vi "Initialize.vi"(8 "error in (no error)":errorcluster, 9 "settings":T1[](array[typedef]), 10 "Group Configurations":refnum<class "Group Configuration.lvclass">[](array[class]), 11 "Type Converter in":refnum<class "Default Buffer Converter.lvclass">) -> (0 "error out":errorcluster, 3 "Type Converter out":refnum<class "Default Buffer Converter.lvclass">)   [LabVIEW 2017, in "DSF Core.lvlib" / "Default Buffer Converter.lvclass"]
uses:
  Default Buffer Converter.lvclass
  Classes/Configuration/Core/Group/Group Configuration.lvclass
  Typedefs/DSF Settings Info.ctl
  Conversion.ctl
  Conversion Block.ctl
  Typedefs/DSF Data Type.ctl
  Default Buffer Converter.lvclass/Default Buffer Converter.ctl
  Classes/Configuration/Core/Transfer/Transfer Configuration.lvclass
  DSF Core.lvlib
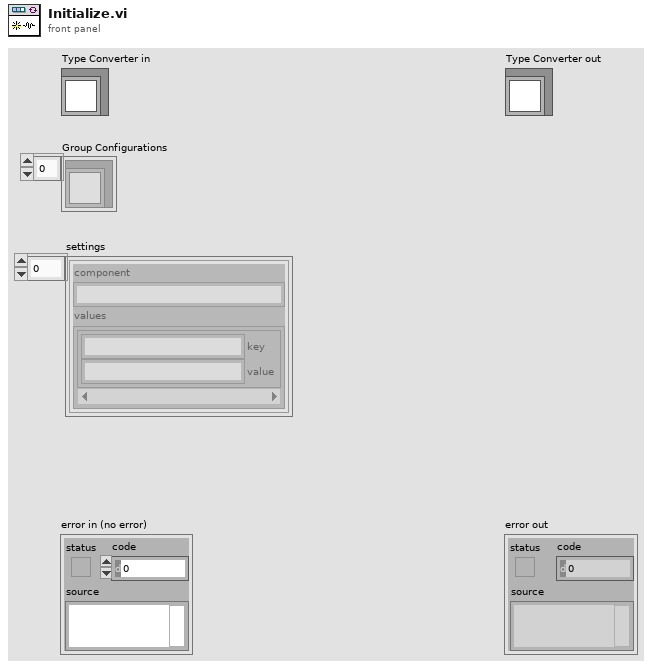
[diagram p1: front panel]
types:
  T1 = typedef "DSF Core.lvlib/DSF Settings Info.ctl" = cluster{"component":string, "values":cluster{"key":string, "value":string}[]}
  T2 = typedef "DSF Core.lvlib/Default Buffer Converter.lvclass/Conversion.ctl" = cluster{"conversion blocks":T3[]}
  T3 = typedef "DSF Core.lvlib/Default Buffer Converter.lvclass/Conversion Block.ctl" = cluster{"engine offset":u64, "engine data type":T4, "string offset":u64, "string data type":T4, "engine byte order":enum16{"big-endian, network order", "native, host order", "little-endian"}, "string byte order":enum16{"big-endian, network order", "native, host order", "little-endian"}, "count":u64}
  T4 = typedef "DSF Core.lvlib/DSF Data Type.ctl" = enum8{"Bool", "SGL", "DBL", "I8", "I16", "I32", "I64", "U8", "U16", "U32", "U64"}
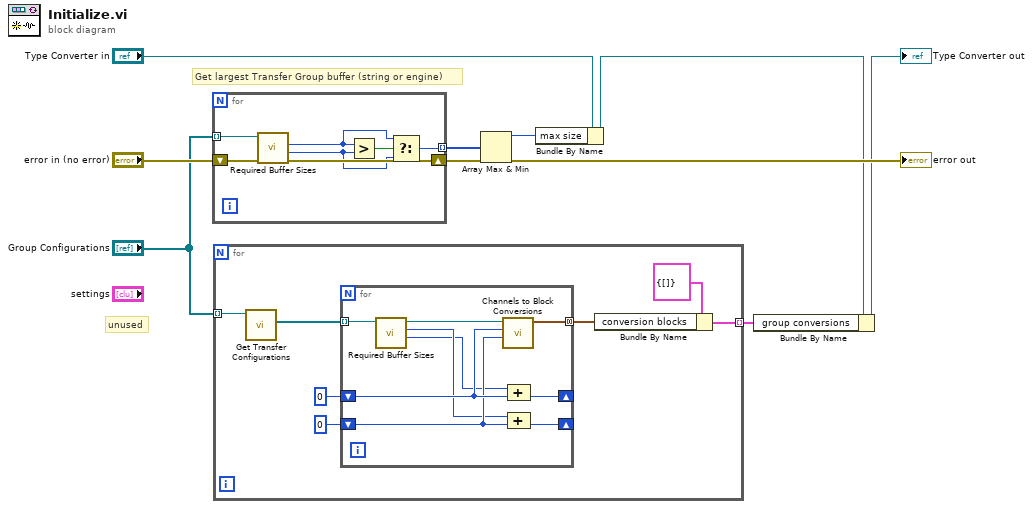
[diagram p0: block diagram]
diagram:
  # "Get largest Transfer Group buffer (string or engine)"
  # "unused"
  n1 = for {
    tunnel: "Group Configurations" -> [w14] mode=indexing
    tunnel: [w15] -> w8 mode=indexing
    shift-right: [w12] -> w9
    shift-left: "error in (no error)" -> [w13]
    n2 = call-dynamic "Required Buffer Sizes.vi"("error in (no error)"=w13, "Group Configuration in"=w14) -> ("error out"=w12:errorcluster, "string size"=w11:u64, "engine size"=w10:u64)  [unwired: 6 in, 1 out]
    n3 = Greater?(x=w10, y=w11) -> (0:w16:bool)
    n4 = Select(t=w10, s=w16, f=w11) -> (s? t:f=w15:u64)
  }
  "error out" <- w9
  n5 = for {
    tunnel: "Group Configurations" -> [w18] mode=indexing
    tunnel: [w21] -> w6 mode=indexing
    n6 = call "Get Transfer Configurations.vi"("Group Configuration in"=w18) -> ("Transfer Configurations"=w17:refnum<class "Transfer Configuration.lvclass">[])  [unwired: 8 in, 2 out]
    n7 = for {
      tunnel: w17 -> [w27] mode=indexing
      tunnel: [w32] -> w22 mode=concatenating
      shift-right: [w31] -> _
      shift-left: u64 0 ("engine buffer size") -> [w29]
      shift-right: [w30] -> _
      shift-left: u64 0 ("engine buffer size") -> [w28]
      n8 = call-dynamic "Required Buffer Sizes.vi"("Transfer Configuration in"=w27) -> ("string size"=w24:u64, "engine size"=w25:u64, "Transfer Configuration out"=w26:refnum<class "Transfer Configuration.lvclass">)  [unwired: 7 in, 1 out]
      n9 = call "Channels to Block Conversions.vi"("initial engine buffer offset"=w28, "initial string buffer offset"=w29, "Transfer Configuration"=w26) -> ("Transfer conversion descriptors"=w32:T3[])  [unwired: 8 in]
      n10 = Compound Arithmetic op=ADD(w24, w29) -> (w31:u64)
      n11 = Compound Arithmetic op=ADD(w25, w28) -> (w30:u64)
    }
    n12 = Bundle By Name(cluster=T2 {"conversion blocks"=[]} ("conversion"), "conversion blocks"=w22) -> (w21:T2)
  }
  n13 = Array Max & Min(array=w8) -> (max value=w1:u64)  [unwired: 3 out]
  n14 = Bundle By Name(cluster="Type Converter in", "max size"=w1) -> (w2:refnum<class "Default Buffer Converter.lvclass">)
  n15 = Bundle By Name(cluster=w2, "group conversions"=w6) -> (→"Type Converter out":refnum<class "Default Buffer Converter.lvclass">)
